vi "Run.vi"(8 "error in":errorcluster, 10 "Execution Plan":T1={"Exe Path"=path "", "Args"=[], "Timeout"=-1}, 11 "IProcess Executor in":refnum<class "IProcess Executor.lvclass">) -> (0 "error out":errorcluster, 3 "IProcess Executor out":refnum<class "IProcess Executor.lvclass">)   [LabVIEW 2025, in "IProcess Executor.lvclass"]
doc: "Run executes an external process as defined by an Execution Plan.\n\nThe method starts the specified executable with the provided command-line arguments and applies the configured timeout behavior. If the timeout is set to -1, the method waits indefinitely for the process to terminate; otherwise, it waits up to the specified number of seconds and reports an error if the process does not complete in time."
uses:
  IProcess Executor.lvclass
  Type Definitions/Execution Plan--cluster.ctl
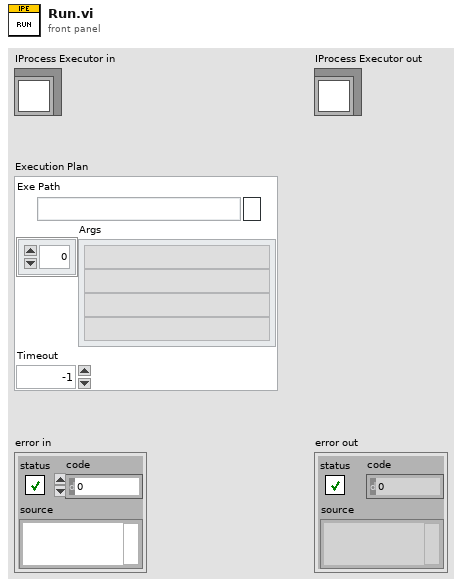
[diagram p1: front panel]
types:
  T1 = typedef "Execution Plan--cluster.ctl" = cluster{"Exe Path":path, "Args":string[], "Timeout":i32}
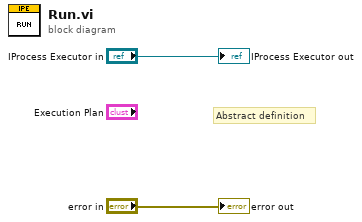
[diagram p0: block diagram]
diagram:
  # "Abstract definition"
  "error out" <- "error in"
  "IProcess Executor out" <- "IProcess Executor in"
